vi "Test2_5.vi"(0 "Instrument VISA in":T1={"AWG VISA"="AGTMY51400121", "Oscilloscope  VISA "="labosc4", "Integration Board IP"="172.16.7.43", "connection ID"=refnum, "report out"=refnum, "report file path"=path "C:/CTA/LevelTriggerBoardTest/TestsData/sumtrigger_delay/tmp"}, 1 "Att minims":i32[](array[numeric]), 2 "Report Enable":bool=TRUE, 5 "Att Calibration":i32[](array[numeric]), 7 "channels":i32[](array[numeric]), 9 "Cycles Burst":i32=10000, 11 "error in":errorcluster, 12 "voltages":dbl[](array[numeric]), 13 "L1 version":bool) -> (4 "Instrument VISA out":T1, 6 "Clipping":dbl[][](array[numeric]), 8 "XY Graph":cluster{"Y":dbl[], "Y":dbl[]}[](graph), 15 "error out":errorcluster)   [LabVIEW 2009]
uses:
  <vilib>/Utility/NIReport.llb/NI_report.lvclass
  <vilib>/Analysis/NI_AALPro.lvlib
  <instrlib>/Agilent 81150/Agilent 81150.lvlib
panel:
  out "XY Graph 2":cluster{"Y":dbl[], "Y":dbl[]}[](graph)
  out "report file path":path=path "D:/CTA/LevelTriggerBoardTest/TestsData/sumtrigger_delay"
  out "IPR_Address":i32
  out "L1 Address":i32=17
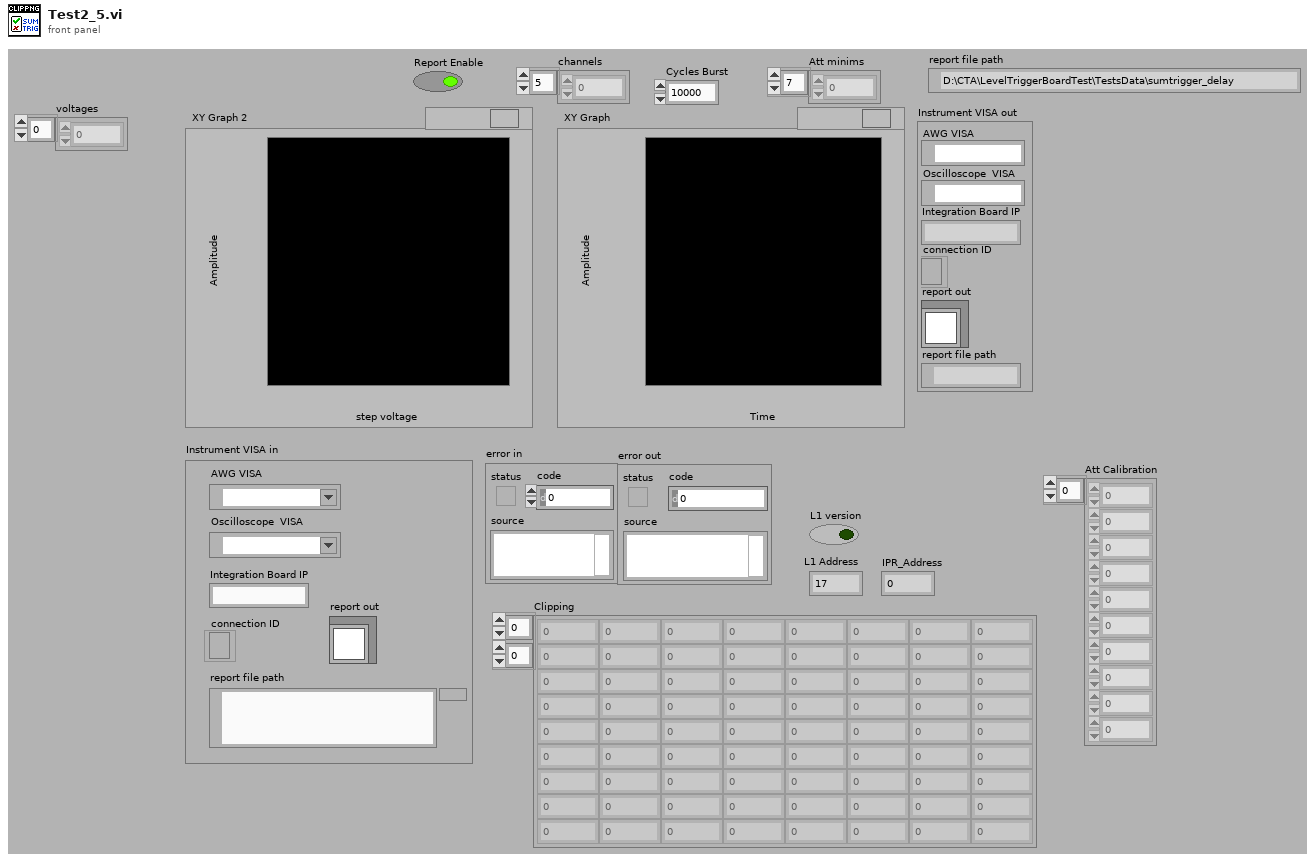
[diagram p1: front panel]
types:
  T1 = cluster{"AWG VISA":refnum<visa-resource-name>, "Oscilloscope  VISA ":refnum<visa-resource-name>, "Integration Board IP":string, "connection ID":refnum<k5>, "report out":refnum<class "NI_report.lvclass">, "report file path":path}
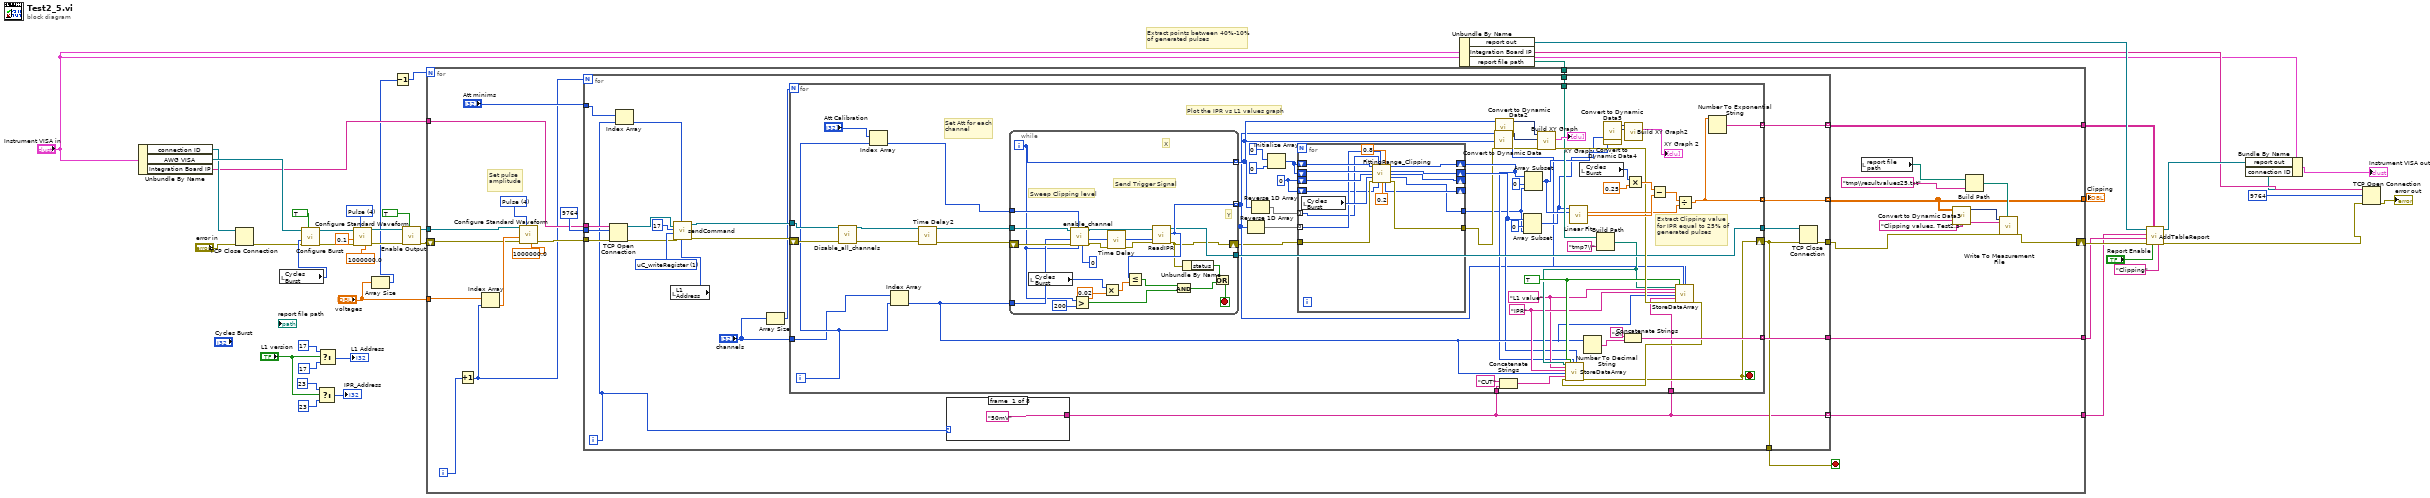
[diagram p0: block diagram]
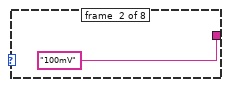
[diagram p2: hidden frame]
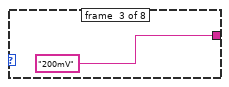
[diagram p3: hidden frame]
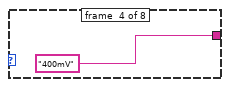
[diagram p4: hidden frame]
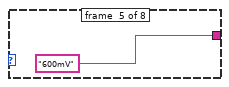
[diagram p5: hidden frame]
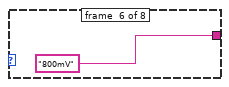
[diagram p6: hidden frame]
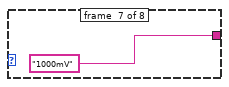
[diagram p7: hidden frame]
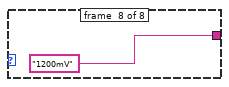
[diagram p8: hidden frame]
diagram:
  w43 = u16 4 items=["Sine", "Square", "Ramp Up", "Ramp Down", "Pulse", "Noise", "DC"] ("Waveform (0: Sine)")
  # "Extract points between 40%-10% of generated pulses"
  n1 = Unbundle By Name("Instrument VISA in") -> ("connection ID"=w17:refnum<k5>, "AWG VISA"=w34:refnum<visa-resource-name>, "Integration Board IP"=w9:string)
  n2 = TCP Close Connection(connection ID=w17, error in (no error)="error in") -> (error out=w15:errorcluster)  [unwired: 1 in, 1 out]
  n3 = local read "Cycles Burst"() -> (w35:i32)
  n4 = call <instrlib>:"Configure Burst.vi"("Enable Burst (F: Disable)"=TRUE, "error in (no error)"=w15, "Burst Count (2)"=w35, "VISA resource name"=w34) -> ("error out"=w40:errorcluster, "VISA resource name out"=w41:refnum<visa-resource-name>)  [unwired: 6 in]
  n5 = Select(t=23 ("Address"), s="L1 version", f=23 ("Address")) -> (s? t:f=→"IPR_Address":i32)
  n6 = Select(t=17 ("Address"), s="L1 version", f=17 ("Address")) -> (s? t:f=→"L1 Address":i32)
  n7 = call <instrlib>:"Configure Standard Waveform.vi"("Frequency (1000.0 Hz)"=1000000.0, "Waveform (0: Sine)"=w43, "error in (no error)"=w40, "Amplitude (1.0 Vpp)"=0.1, "VISA resource name"=w41) -> ("error out"=w39:errorcluster, "VISA resource name out"=w38:refnum<visa-resource-name>)  [unwired: 5 in]
  n8 = Array Size(array="voltages") -> (size(s)=w1:i32)
  n9 = Decrement(x=w1) -> (x-1=w2:i32)
  n10 = call <instrlib>:"Enable Output.vi"("Enable Output (T: Enable)"=TRUE, "error in (no error)"=w39, "VISA resource name"=w38) -> ("error out"=w14:errorcluster, "VISA resource name out"=w33:refnum<visa-resource-name>)  [unwired: 7 in]
  n11 = Unbundle By Name("Instrument VISA in") -> ("report out"=w31:refnum<class "NI_report.lvclass">, "Integration Board IP"=w12:string, "report file path"=w6:path)
  n12 = for {
    N: w2 -> [_]
    shift-right: [w50] -> w32
    shift-left: w14 -> [w66]
    tunnel: w33 -> [w65]
    tunnel: [w49] -> w5
    tunnel: [w64] -> w27
    tunnel: [w57] -> w25
    tunnel: [w63] -> w26
    tunnel: w9 -> [w61]
    tunnel: w6 -> [w58]
    tunnel: "voltages" -> [w48]
    i -> [w46]
    stop <- w59 stop-if-true
    w68 = u16 4 items=["Sine", "Square", "Ramp Up", "Ramp Down", "Pulse", "Noise", "DC"] ("Waveform (0: Sine)")
    # "Set pulse amplitude"
    n13 = Increment(x=w46) -> (x+1=w45:i32)
    n14 = Index Array(array=w48, index=w45) -> (element=w67:dbl)
    n15 = call <instrlib>:"Configure Standard Waveform.vi"("Frequency (1000.0 Hz)"=1000000.0, "Waveform (0: Sine)"=w68, "error in (no error)"=w66, "Amplitude (1.0 Vpp)"=w67, "VISA resource name"=w65) -> ("error out"=w60:errorcluster)  [unwired: 5 in, 1 out]
    n16 = for {
      N: w45 -> [_]
      tunnel: [w92] -> w49 mode=indexing
      tunnel: [w91] -> w64 mode=indexing
      tunnel: [w90] -> w63
      tunnel: u16 9764 ("remote port or service name") -> [w89]
      tunnel: w61 -> [w88]
      tunnel: w60 -> [w87]
      tunnel: [w78] -> w59
      tunnel: [w77] -> w51
      tunnel: w58 -> [w75]
      tunnel: [w72] -> w57 mode=indexing
      tunnel: "Att minims" -> [w71]
      i -> [w70]
      w85 = u16 1 items=["sendCommand"=9, "FPGA_writeRegister"=3, "FPGA_readRegister"=2, "uC_writeRegister"=1, "uC_readRegister"=0] ("Action")
      n17 = TCP Open Connection(address=w88, remote port or service name=w89, error in (no error)=w87) -> (connection ID=w81:refnum<k5>, error out=w82:errorcluster)  [unwired: 2 in]
      n18 = Index Array(array=w71, index=w70) -> (element=w79:i32)
      n19 = local read "L1 Address"() -> (w86:i32)
      n20 = call "sendCommand.vi"("Address"=w86, "Data"=w79, "error in"=w82, "Action"=w85, "id_in"=17 ("id"), "connection ID"=w81) -> ("error out"=w83:errorcluster, "connection ID out"=w80:refnum<k5>)  [unwired: 1 in, 3 out]
      n21 = Array Size(array="channels") -> (size(s)=w73:i32)
      n22 = case shown="0, Default" w70 {
        tunnel: ["50mV" ("regular expression") "100mV" ("regular expression") "200mV" ("regular expression") "400mV" ("regular expression") "600mV" ("regular expression") "800mV" ("regular expression") "1000mV" ("regular expression") "1200mV" ("regular expression")] -> w72
        frame #0 {
        }
        frame #1 {
        }
        frame #2 {
        }
        frame #3 {
        }
        frame #4 {
        }
        frame #5 {
        }
        frame #6 {
        }
        frame #7 {
        }
      }
      n23 = for {
        N: w73 -> [_]
        tunnel: [w146] -> w92 mode=indexing
        shift-right: [w128] -> w78
        shift-left: w83 -> [w137]
        tunnel: w80 -> [w136]
        tunnel: [w145] -> w91 mode=indexing
        tunnel: [w142] -> w90 mode=indexing
        tunnel: [w140] -> w76
        tunnel: w75 -> [w139]
        tunnel: w72 -> [w126]
        tunnel: "channels" -> [w114]
        tunnel: w72 -> [w125]
        i -> [w116]
        stop <- w128 stop-if-true
        w102 = 0 ("Array Pointer out")
        w131 = "IPR" ("Y Signal Name")
        w130 = "L1 value" ("X Signal Name")
        w133 = TRUE ("Save test data")
        # "Set Att for each channel"
        # "Extract Clipping value for IPR equal to 25% of generated pulses"
        # "Plot the IPR vs L1 values graph"
        n24 = call "Disable_all_channels.vi"("error in"=w137, "connection ID"=w136) -> ("error out"=w123:errorcluster, "connection ID out"=w134:refnum<k5>)  [unwired: 7 in, 1 out]
        n25 = Index Array(array="Att Calibration", index=w116) -> (element=w135:i32)
        n26 = Index Array(array=w114, index=w116) -> (element=w115:i32)
        n27 = call "Time Delay2"("error in (no error)"=w123) -> ("error out"=w122:errorcluster)  [unwired: 10 in]
        n28 = while {
          tunnel: [w192] -> w110 mode=indexing
          tunnel: [w184] -> w111 mode=indexing
          shift-right: [w175] -> w105
          shift-left: w122 -> [w188]
          tunnel: [w191] -> w140
          tunnel: w135 -> [w189]
          tunnel: w134 -> [w186]
          tunnel: w115 -> [w185]
          i -> [w184]
          stop <- w193 stop-if-true
          # "Sweep Clipping level"
          # "Send Trigger Signal"
          # "Y"
          # "X"
          n29 = local read "Cycles Burst"() -> (w194:i32)
          n30 = call "enable_channel.vi"("Delay"=0, "V clip"=w184, "V att"=w189, "error in"=w188, "Channel"=w185, "connection ID"=w186) -> ("error out"=w182:errorcluster, "id_out"=w177:i32, "connection ID out"=w190:refnum<k5>)  [unwired: 3 in]
          n31 = Greater?(x=w184, y=200) -> (0:w179:bool)
          n32 = Multiply(x=w194, y=0.02) -> (x*y=w195:dbl)
          n33 = call "Time Delay"("error in (no error)"=w182) -> ("error out"=w181:errorcluster)  [unwired: 10 in]
          n34 = call "ReadIPR.vi"("error in"=w181, "id_in"=w177, "connection ID"=w190) -> ("error out"=w175:errorcluster, "IPR value"=w192:i32, "connection ID out"=w191:refnum<k5>)  [unwired: 6 in]
          n35 = Less Or Equal?(x=w192, y=w195) -> (x <= y?=w180:bool)
          n36 = And(x=w180, y=w179) -> (x .and. y?=w178:bool)
          n37 = Unbundle By Name(w175) -> ("status"=w176:bool)
          n38 = Or(x=w176, y=w178) -> (x .or. y?=w193:bool)
        }
        n39 = Reverse 1D Array(array=w110) -> (reversed array=w106:i32[])
        n40 = Reverse 1D Array(array=w111) -> (reversed array=w103:i32[])
        n41 = Initialize Array(0 ("element"), 0 ("dimension size")) -> (w107:i32[])
        n42 = for {
          shift-right: [w174] -> w113
          shift-left: w107 -> [w171]
          shift-right: [w173] -> w112
          shift-left: w107 -> [w172]
          tunnel: w106 -> [w165] mode=indexing
          shift-right: [w169] -> _
          shift-left: w102 -> [w170]
          tunnel: w105 -> [w168]
          tunnel: [w167] -> w104
          tunnel: w103 -> [w164] mode=indexing
          shift-right: [w160] -> _
          shift-left: w102 -> [w161]
          tunnel: [w159] -> w101
          n43 = local read "Cycles Burst"() -> (w166:i32)
          n44 = call "FittingRange_Clipping.vi"("Array in (X)"=w172, "L0 DAC"=w164, "IPR"=w165, "upper limit"=0.8, "Array in (Y)"=w171, "Array Pointer in"=w170, "Cycles Burst"=w166, "error in"=w168, "State machine"=w161, "lower limit"=0.2) -> ("Array out (X)"=w173:i32[], "Array out (Y)"=w174:i32[], "Array Pointer out"=w169:i32, "N_Array Elements"=w159:i32, "State machine"=w160:i32, "error out"=w167:errorcluster)
        }
        n45 = call "Convert to Dynamic Data"("Array"=w110) -> ("Dynamic Data Type"=w157:dynamicdata)  [unwired: 3 in]
        n46 = call "Convert to Dynamic Data2"("Array"=w111) -> ("Dynamic Data Type"=w156:dynamicdata)  [unwired: 3 in]
        n47 = Concatenate Strings("CUT" ("string"), w125) -> (w127:string)
        n48 = Array Subset(array=w113, index=0, length=w101) -> (w117:i32[])
        n49 = Array Subset(array=w112, index=0, length=w101) -> (w118:i32[])
        n50 = call "Build XY Graph"("error in (no error)"=w104, "Y Input"=w157, "X Input"=w156) -> ("error out"=w141:errorcluster, "XY Graph"=→"XY Graph":cluster{"Y":dbl[], "Y":dbl[]}[])  [unwired: 7 in]
        n51 = call <vilib>:"Linear Fit.vi"("Y"=w117, "X"=w118) -> ("slope"=w148:dbl, "intercept"=w150:dbl)  [unwired: 9 in, 3 out]
        n52 = local read "Cycles Burst"() -> (w153:i32)
        n53 = Number To Decimal String(number=w115) -> (decimal integer string=w143:string)  [unwired: 1 in]
        n54 = Build Path(base path=w139, name or relative path="tmp7\\") -> (appended path=w132:path)
        n55 = call "Convert to Dynamic Data4"("Array"=w118) -> ("Dynamic Data Type"=w121:dynamicdata)  [unwired: 3 in]
        n56 = call "Convert to Dynamic Data5"("Array"=w117) -> ("Dynamic Data Type"=w120:dynamicdata)  [unwired: 3 in]
        n57 = Concatenate Strings("ch" ("string"), w143) -> (w142:string)
        n58 = call "Build XY Graph2"("Y Input"=w120, "X Input"=w121) -> ("XY Graph"=→"XY Graph 2":cluster{"Y":dbl[], "Y":dbl[]}[])  [unwired: 8 in, 1 out]
        n59 = Multiply(x=w153, y=0.25) -> (x*y=w151:dbl)
        n60 = Subtract(x=w151, y=w150) -> (x-y=w149:dbl)
        n61 = call "StoreDataArray.vi"("Base path"=w132, "X Signal Name"=w130, "Y Signal Name"=w131, "Channel number"=w115, "Si"=w126, "error in"=w141, "Save test data"=w133, "X Array"=w111, "Y Array"=w110) -> ("error out"=w129:errorcluster)  [unwired: 10 in]
        n62 = call "StoreDataArray.vi"("Base path"=w132, "X Signal Name"=w130, "Y Signal Name"=w131, "Channel number"=w115, "Si"=w127, "error in"=w129, "Save test data"=w133, "X Array"=w112, "Y Array"=w113) -> ("error out"=w128:errorcluster)  [unwired: 10 in]
        n63 = Divide(x=w149, y=w148) -> (x/y=w146:dbl)
        n64 = Number To Exponential String(number=w146) -> (E-format string=w145:string)  [unwired: 3 in]
      }
      n65 = TCP Close Connection(connection ID=w76, error in (no error)=w78) -> (error out=w77:errorcluster)  [unwired: 1 in, 1 out]
    }
    n66 = local read "report file path"() -> (w56:path)
    n67 = call "Convert to Dynamic Data3"("2D Array"=w49) -> ("Dynamic Data Type"=w52:dynamicdata)  [unwired: 3 in]
    n68 = Build Path(base path=w56, name or relative path="tmp\\resultvalues25.txt") -> (appended path=w54:path)
    n69 = call "Write To Measurement File"("Signals"=w52, "error in (no error)"=w51, "Filename"=w54, "Comment"="Clipping values. Test2.5") -> ("error out"=w50:errorcluster)  [unwired: 13 in, 2 out]
  }
  "Clipping" <- w5
  n70 = call "AddTableReport.vi"("Table title"="Clipping", "Report Enable"="Report Enable", "Data"=w27, "error in"=w32, "Columns"=w26, "Rows"=w25, "report in"=w31) -> ("error out"=w4:errorcluster, "report out"=w30:refnum<class "NI_report.lvclass">)  [unwired: 3 in]
  n71 = TCP Open Connection(address=w12, remote port or service name=u16 9764, error in (no error)=w4) -> (connection ID=w10:refnum<k5>, error out=→"error out":errorcluster)  [unwired: 2 in]
  n72 = Bundle By Name(cluster="Instrument VISA in", "report out"=w30, "connection ID"=w10) -> (→"Instrument VISA out":T1)
